vi "1_08.vi"() -> ()   [LabVIEW 2013]
uses:
  <vilib>/sound2/lvsound2.llb/Sound Data Format.ctl
  <vilib>/sound2/lvsound2.llb/Sound Input Read (DBL).vi
panel:
  out "Boolean":bool
  in  "Umbral":dbl
  in  "stop":bool
  out "Waveform Graph":dbl[](graph)
  in  "Buffer de Lectura":dbl=1000.0
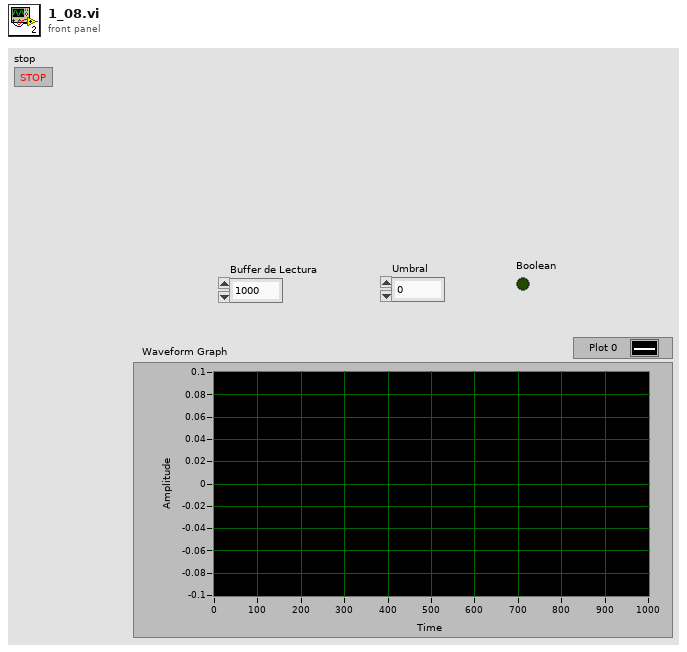
[diagram p1: front panel]
types:
  T1 = typedef "Sound Data Format.ctl" = cluster{"sample rate (S/s)":dbl, "number of channels":i32, "bits per sample":i32}
  T2 = typedef "Sound Input Task ID.ctl" = u32
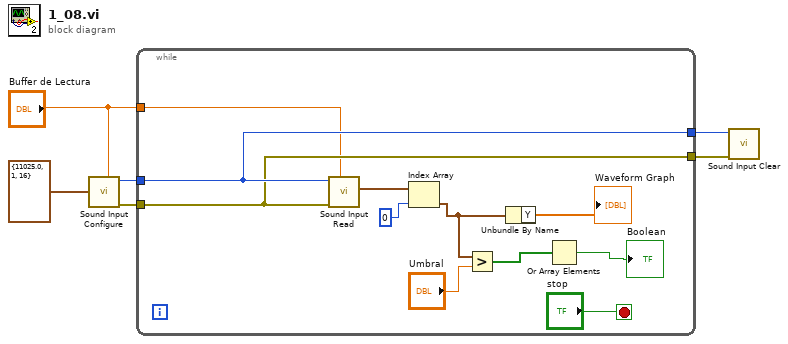
[diagram p0: block diagram]
diagram:
  n1 = call <vilib>:"Sound Input Configure.vi"("number of samples/ch"="Buffer de Lectura", "sound format"=T1 {"sample rate (S/s)"=11025.0, "number of channels"=1, "bits per sample"=16}) -> ("error out"=w4:errorcluster, "task ID"=w5:T2)  [unwired: 8 in]
  n2 = while {
    tunnel: w5 -> [w17]
    tunnel: w4 -> [w16]
    tunnel: [w17] -> w3
    tunnel: [w16] -> w2
    tunnel: "Buffer de Lectura" -> [w15]
    stop <- "stop" stop-if-true
    n3 = call-poly <vilib>:"Sound Input Read.vi"("number of samples/ch"=w15, "error in (no error)"=w16, "task ID"=w17) -> ("data"=w14:waveform(dbl)[])  [unwired: 6 in, 2 out]
    n4 = Index Array(array=w14, index=0) -> (element=w9:waveform(dbl))
    n5 = Greater?(x=w9, y="Umbral") -> (0:w8:bool[])
    n6 = Unbundle By Name(w9) -> ("Y"=→"Waveform Graph":dbl[])
    n7 = Or Array Elements(Boolean array=w8) -> (logical OR=→"Boolean":bool)
  }
  n8 = call <vilib>:"Sound Input Clear.vi"("error in (no error)"=w2, "task ID"=w3) -> ()  [unwired: 9 in, 1 out]
